vi "Pressure_Multiplexer.vi"() -> (0 "DAQ Error":errorcluster)   [LabVIEW 2020]
uses:
  <vilib>/Instr/_visa.llb/VISA Find Search Mode.ctl
  Globals/Meas_global.vi
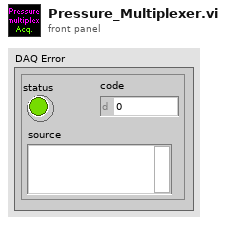
[diagram p1: front panel]
types:
  T1 = typedef "Analysis_info_cluster.ctl" = cluster{"Colour":u32, "Inst type":T2, "Inst name":string, "Symbol":string, "Code name":string, "Extra Info":string, "Inst Array":T3, "Extra Titles":string[], "Extra Values":string[], "U":dbl, "u^2":dbl, "u^3":dbl, "u^4":dbl, "Skew_u":dbl, "Kurt_u":dbl, "Sd Error in Mean":dbl, "% u'/U":dbl, "X":dbl, "Y":dbl, "Z":dbl, "Timescale integral Estimate":dbl, "Sd Error in Variance":dbl, "Calib File":path, "Calib Constants":dbl[], "Output Position":bool, "Stats":enum16{"None", "Basic", "Full"}, "Av Sampling Rate":dbl, "Av No of Samples":dbl, "Total Meas Time (s)":dbl, "ADAM Ch Name":string, "Max value":dbl, "Min value":dbl, "Req Sample Rate Hz":dbl, "Sync Delay Time (s)":dbl, "Ch No":i16, "Device":string, "Use Latest Calib":bool, "Port":string, "Metadata Ch Names":string[], "Metadata Ch Values":string[], "Label":string}
  T2 = typedef "Inst_type.ctl" = enum16{"Raw voltage", "Raw with zero offsetting", "Propeller anemometer", "Pressure Transducer", "Pitot-static tube", "Hot wire", "Cross wire 1", "Cross wire 2", "Generic Linear", "Generic Polynomial", "Generic BackPoly", "Fast FID", "Thermocouple", "Cold wire", "Pulsed Wire", "LDA Vel", "LDA Tran time", "LDA Arr time", "Microphone"}
  T3 = typedef "Instrument_Array.ctl" = enum16{"PWA", "LDA", "Analogue"}
  T4 = typedef "Device ID port info.ctl" = cluster{"Ch No":i16[], "Req Sampling Rate":dbl[], "Port":string, "Index":i32[]}
  T5 = typedef "Setup.ctl" = enum16{"Run Program", "Show Setup", "Save Current Setup", "Setup Front Panel"}
  T6 = typedef "VISA Find Search Mode.ctl" = u32
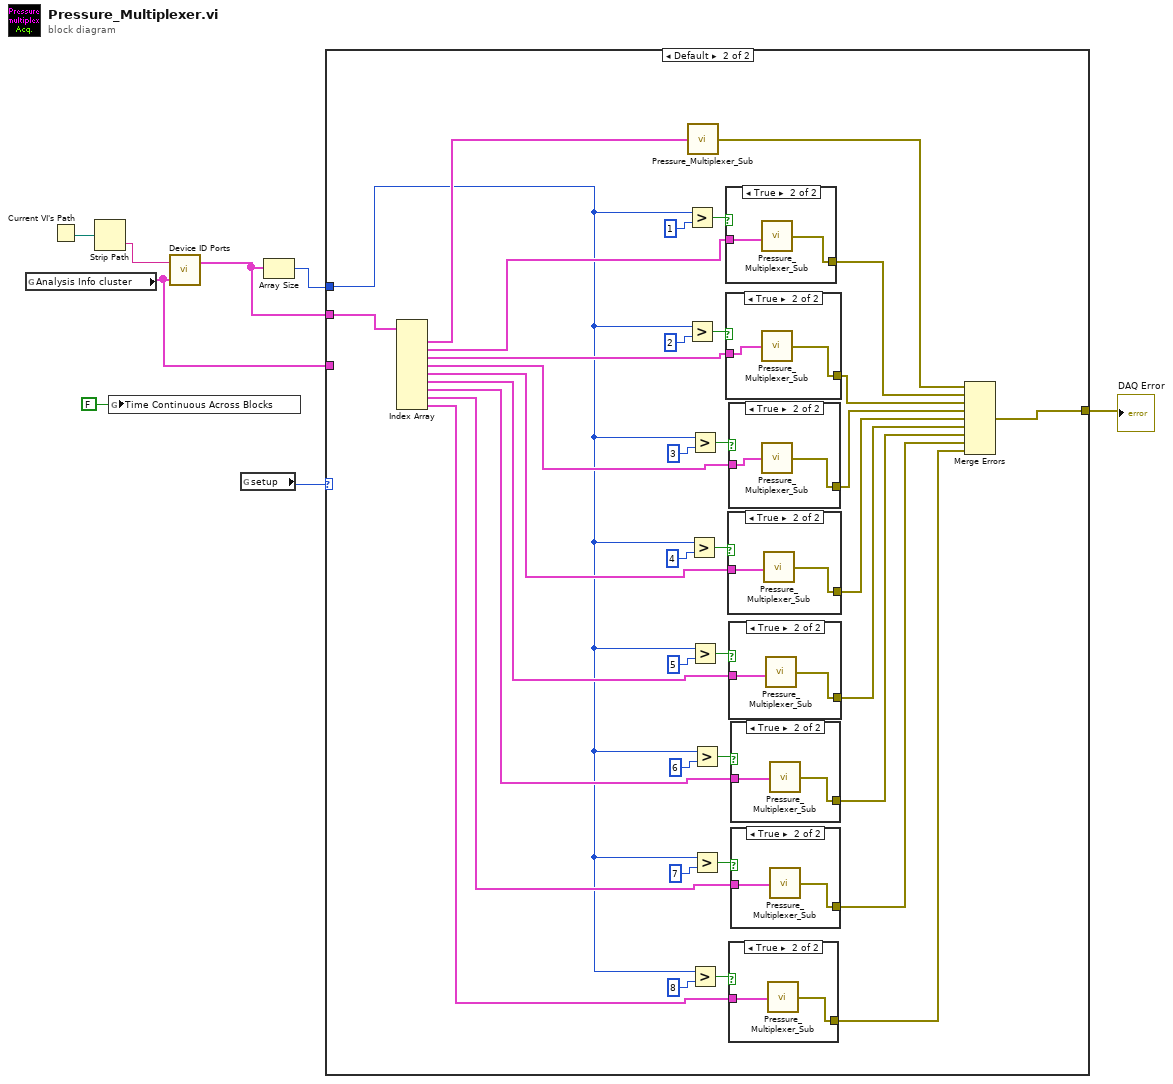
[diagram p0: block diagram]
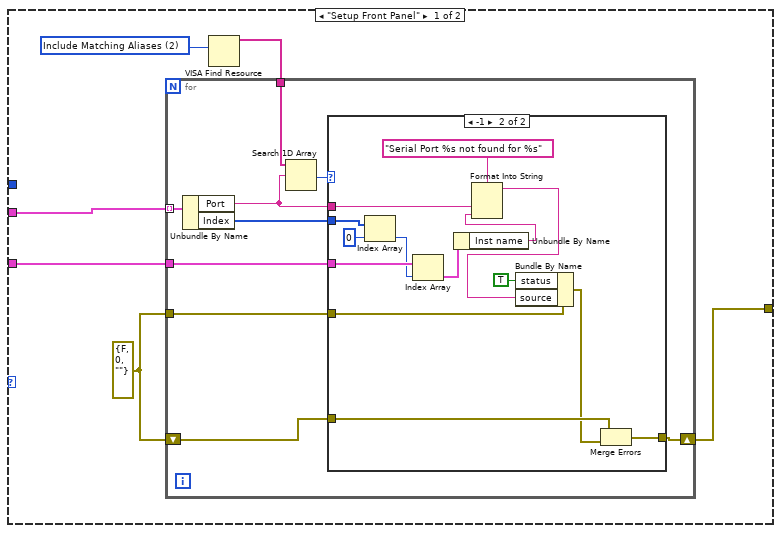
[diagram p2: hidden frame]
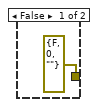
[diagram p4: hidden frame]
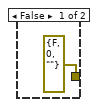
[diagram p5: hidden frame]
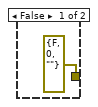
[diagram p6: hidden frame]
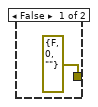
[diagram p7: hidden frame]
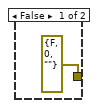
[diagram p8: hidden frame]
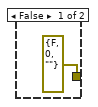
[diagram p9: hidden frame]
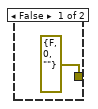
[diagram p10: hidden frame]
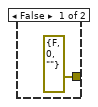
[diagram p11: hidden frame]
diagram:
  n1 = global read "Meas_global.vi" "Analysis Info cluster"() -> (w8:T1[])
  n2 = Current VI's Path() -> (path=w5:path)
  n3 = Strip Path(path=w5) -> (name=w6:string)  [unwired: 1 out]
  n4 = global write "Meas_global.vi" "Time Continuous Across Blocks"(FALSE ("Time Continuous across Blocks")) -> ()
  n5 = call "Device ID Ports.vi"("Analysis Info cluster"=w8, "Device ID"=w6) -> ("Device port info"=w7:T4[])  [unwired: 1 out]
  n6 = global read "Meas_global.vi" "setup"() -> (w4:T5)
  n7 = Array Size(array=w7) -> (size(s)=w3:i32)
  n8 = case shown="Default" w4 {
    tunnel: w7 -> [w14 w75]
    tunnel: w3 -> [_ w39]
    tunnel: [w13 w50] -> w2
    tunnel: w8 -> [w9 _]
    frame "Setup Front Panel" {
      w12 = T6 2 items=["Canonical Names Only"=0, "Aliases Only"=1, "Include Matching Aliases"=2, "Include All Aliases"=4] ("Search Mode")
      w10 = errorcluster {"status"=FALSE, "code"=0, "source"=""} ("error IO")
      n9 = VISA Find Resource(10:w12) -> (3:w11:string[])  [unwired: 1 in, 3 out]
      n10 = for {
        tunnel: w14 -> [w23] mode=indexing
        shift-right: [w21] -> w13
        shift-left: w10 -> [w22]
        tunnel: w11 -> [w20]
        tunnel: w10 -> [w18]
        tunnel: w9 -> [w15]
        n11 = Unbundle By Name(w23) -> ("Port"=w17:string, "Index"=w16:i32[])
        n12 = Search 1D Array(1D array=w20, element=w17) -> (index of element=w19:i32)  [unwired: 1 in]
        n13 = case shown="-1" w19 {
          tunnel: w22 -> [w24 w37]
          tunnel: [w24 w38] -> w21
          tunnel: w18 -> [_ w34]
          tunnel: w17 -> [_ w33]
          tunnel: w16 -> [_ w31]
          tunnel: w15 -> [_ w29]
          frame 0, Default {
          }
          frame -1 {
            n14 = Index Array(array=w31, index=0) -> (element=w28:i32)
            n15 = Index Array(array=w29, index=w28) -> (element=w27:T1)
            n16 = Unbundle By Name(w27) -> ("Inst name"=w26:string)
            n17 = Format Into String(format string="Serial Port %s not found for %s", w33, w26) -> (resulting string=w25:string)  [unwired: 2 in, 1 out]
            n18 = Bundle By Name(cluster=w34, "status"=TRUE, "source"=w25) -> (w35:errorcluster)
            n19 = Merge Errors(w37, w35) -> (w38:errorcluster)
          }
        }
      }
    }
    frame Default {
      n20 = Index Array(array=w75) -> (element #1=w49:T4, element #2=w62:T4, element #3=w61:T4, element #4=w60:T4, element #5=w59:T4, element #6=w58:T4, element #7=w57:T4, element #8=w45:T4, element #9=w40:T4)  [unwired: 9 in]
      n21 = Greater?(x=w39, y=1) -> (0:w73:bool)
      n22 = Greater?(x=w39, y=2) -> (0:w72:bool)
      n23 = call "Pressure_Multiplexer_Sub.vi"("Single Pres Multiplexer"=w49) -> ("DAQ Error"=w48:errorcluster)
      n24 = Greater?(x=w39, y=4) -> (0:w68:bool)
      n25 = Greater?(x=w39, y=3) -> (0:w69:bool)
      n26 = Greater?(x=w39, y=5) -> (0:w65:bool)
      n27 = Greater?(x=w39, y=8) -> (0:w43:bool)
      n28 = Greater?(x=w39, y=6) -> (0:w64:bool)
      n29 = Greater?(x=w39, y=7) -> (0:w46:bool)
      n30 = case shown="True" w73 {
        tunnel: w62 -> [_ w99]
        tunnel: [errorcluster {"status"=FALSE, "code"=0, "source"=""} ("DAQ Error") w98] -> w56
        frame False {
        }
        frame True {
          n31 = call "Pressure_Multiplexer_Sub.vi"("Single Pres Multiplexer"=w99) -> ("DAQ Error"=w98:errorcluster)
        }
      }
      n32 = case shown="True" w72 {
        tunnel: w61 -> [_ w96]
        tunnel: [errorcluster {"status"=FALSE, "code"=0, "source"=""} ("DAQ Error") w95] -> w55
        frame False {
        }
        frame True {
          n33 = call "Pressure_Multiplexer_Sub.vi"("Single Pres Multiplexer"=w96) -> ("DAQ Error"=w95:errorcluster)
        }
      }
      n34 = case shown="True" w68 {
        tunnel: w59 -> [_ w90]
        tunnel: [errorcluster {"status"=FALSE, "code"=0, "source"=""} ("DAQ Error") w89] -> w53
        frame False {
        }
        frame True {
          n35 = call "Pressure_Multiplexer_Sub.vi"("Single Pres Multiplexer"=w90) -> ("DAQ Error"=w89:errorcluster)
        }
      }
      n36 = case shown="True" w69 {
        tunnel: w60 -> [_ w93]
        tunnel: [errorcluster {"status"=FALSE, "code"=0, "source"=""} ("DAQ Error") w92] -> w54
        frame False {
        }
        frame True {
          n37 = call "Pressure_Multiplexer_Sub.vi"("Single Pres Multiplexer"=w93) -> ("DAQ Error"=w92:errorcluster)
        }
      }
      n38 = case shown="True" w65 {
        tunnel: w58 -> [_ w87]
        tunnel: [errorcluster {"status"=FALSE, "code"=0, "source"=""} ("DAQ Error") w86] -> w52
        frame False {
        }
        frame True {
          n39 = call "Pressure_Multiplexer_Sub.vi"("Single Pres Multiplexer"=w87) -> ("DAQ Error"=w86:errorcluster)
        }
      }
      n40 = case shown="True" w43 {
        tunnel: w40 -> [_ w78]
        tunnel: [errorcluster {"status"=FALSE, "code"=0, "source"=""} ("DAQ Error") w77] -> w41
        frame False {
        }
        frame True {
          n41 = call "Pressure_Multiplexer_Sub.vi"("Single Pres Multiplexer"=w78) -> ("DAQ Error"=w77:errorcluster)
        }
      }
      n42 = case shown="True" w64 {
        tunnel: w57 -> [_ w84]
        tunnel: [errorcluster {"status"=FALSE, "code"=0, "source"=""} ("DAQ Error") w83] -> w51
        frame False {
        }
        frame True {
          n43 = call "Pressure_Multiplexer_Sub.vi"("Single Pres Multiplexer"=w84) -> ("DAQ Error"=w83:errorcluster)
        }
      }
      n44 = case shown="True" w46 {
        tunnel: w45 -> [_ w81]
        tunnel: [errorcluster {"status"=FALSE, "code"=0, "source"=""} ("DAQ Error") w80] -> w44
        frame False {
        }
        frame True {
          n45 = call "Pressure_Multiplexer_Sub.vi"("Single Pres Multiplexer"=w81) -> ("DAQ Error"=w80:errorcluster)
        }
      }
      n46 = Merge Errors(w48, w56, w55, w54, w53, w52, w51, w44, w41) -> (w50:errorcluster)
    }
  }
  "DAQ Error" <- w2
